vi "getData_v3.vi"() -> ()   [LabVIEW 2014]
uses:
  <vilib>/FPGAPlugInAG/cRIO-9039/niLvFpga_Open_cRIO-9039.vi
  <vilib>/Utility/error.llb/Error Cluster From Error Code.vi
  <vilib>/rvi/errors/niLvFpgaAdjustHostInterfaceError.vi
  <vilib>/Utility/file.llb/Write To Spreadsheet File (DBL).vi
  <vilib>/FPGAPlugInAG/cRIO-9039/niLvFpga_Close_cRIO-9039.vi
  <vilib>/rvi/interface/nirviOpenFPGA/nirviOpenFPGA.xnode
  FPGA Bitfiles/test0304_FPGATarget_test92159264_2zD5DwEAdGw.lvbitx
  <vilib>/rvi/interface/nirviMethod/nirviMethod.xnode
  <vilib>/rvi/interface/nirviCloseFPGA/nirviCloseFPGA.xnode
  <vilib>/FPGAPlugInAG/cRIO-9039/niLvFpga_ReadFifo_cRIO-9039.vi
  <vilib>/rvi/errors/niLvFpgaMergeErrorWithErrorCode.vi
panel:
  out "FIFO empty":bool
  out "Elements Remaining":u32=10000
  in  "Time_read":i32=10000
  out "message":string=" INSTRUCTIONS:\r\rNormal Use:  When using subVIs that incorporate the error in/error out (or error I/O) structure, place this handler where you want to inform the user of an error, typically at the end of the I/O data path, as the last action of the program.  If the error in error? is ERROR, the handler creates a message describing the error and its source.  If the type of dialog = 1 (default), the message is displayed to the user, who can only acknowedge it.  If the type = 2, the user can acknowledge the message or abort execution; aborting a program with active I/O is not recommended.  If the type = 0, no message is displayed; this is used to process the error programmatically, and the error out cluster elements are wired to individual terminals for that reason.  \r\rOther Use:\n\r\nlocal testing.  To test the error code of a subVI or function that does not have the error I/O structure, you can wire its error code and a source string to the local error code and error source inputs.  If error in error? indicates no error and error code is not equal to 0, the local code and source are substituted for the error in values, and error? is set TRUE (ERROR)."
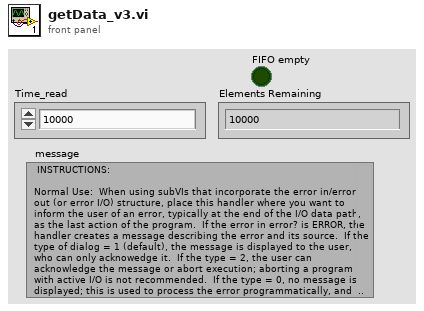
[diagram p1: front panel]
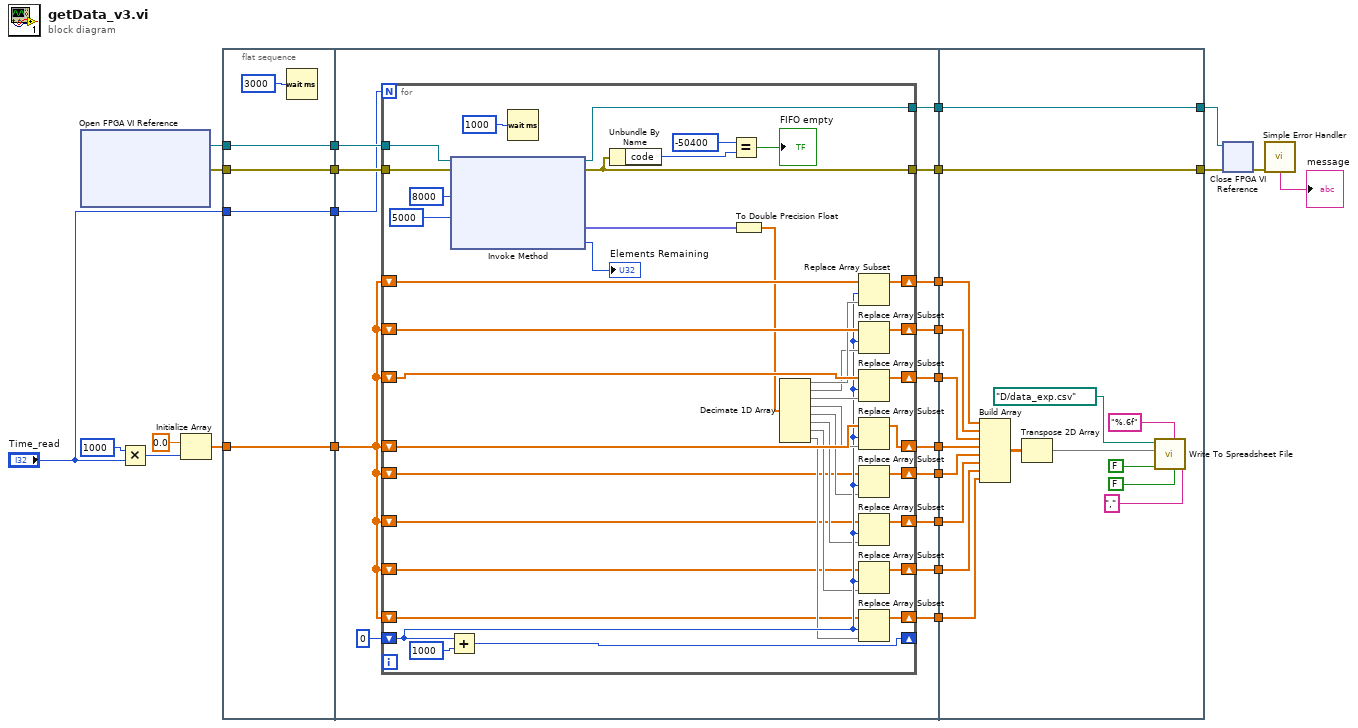
[diagram p0: block diagram]
diagram:
  n1 = xnode "Open FPGA VI Reference"() -> ("FPGA VI Reference Out"=w2:refnum<k20>, "error out"=w1:errorcluster)  [unwired: 2 in]
  n2 = Multiply(x=1000 ("y"), y="Time_read") -> (x*y=w18:i32)
  n3 = Initialize Array(0.0 ("element"), w18) -> (w22:dbl[])
  n4 = flat-sequence {
    tunnel: "Time_read" -> [w27]
    tunnel: w1 -> [w28]
    tunnel: w2 -> [w29]
    tunnel: w22 -> [w30]
    tunnel: [w30] -> w6
    tunnel: [w29] -> w5
    tunnel: [w28] -> w4
    tunnel: [w27] -> w3
    tunnel: [w42] -> w16
    tunnel: [w41] -> w15
    tunnel: [w40] -> w14
    tunnel: [w39] -> w13
    tunnel: [w38] -> w12
    tunnel: [w36] -> w11
    tunnel: [w35] -> w10
    tunnel: [w34] -> w9
    tunnel: [w33] -> w8
    tunnel: [w32] -> w7
    tunnel: w6 -> [w37]
    tunnel: w5 -> [w44]
    tunnel: w4 -> [w43]
    tunnel: w3 -> [w31]
    tunnel: w16 -> [w99]
    tunnel: w15 -> [w98]
    tunnel: w14 -> [w97]
    tunnel: [w102] -> w21
    tunnel: w13 -> [w102]
    tunnel: [w101] -> w20
    tunnel: w12 -> [w101]
    tunnel: w11 -> [w96]
    tunnel: w10 -> [w95]
    tunnel: w9 -> [w93]
    tunnel: w8 -> [w94]
    tunnel: w7 -> [w100]
    frame #0 {
      n5 = Wait (ms)(milliseconds to wait=u32 3000 ("y")) -> ()  [unwired: 1 out]
    }
    frame #1 {
      n6 = for {
        N: w31 -> [_]
        shift-right: [w83] -> _
        shift-left: 0 -> [w69]
        shift-right: [w72] -> w42
        shift-left: w37 -> [w81]
        shift-right: [w71] -> w41
        shift-left: w37 -> [w80]
        shift-right: [w70] -> w40
        shift-left: w37 -> [w79]
        shift-right: [w73] -> w32
        shift-left: w37 -> [w82]
        tunnel: w44 -> [w53]
        tunnel: w43 -> [w52]
        tunnel: [w48] -> w39
        tunnel: [w49] -> w38
        shift-right: [w63] -> w36
        shift-left: w37 -> [w64]
        shift-right: [w61] -> w35
        shift-left: w37 -> [w62]
        shift-right: [w60] -> w33
        shift-left: w37 -> [w59]
        shift-right: [w57] -> w34
        shift-left: w37 -> [w58]
        n7 = Add(x=w69, y=1000) -> (x+y=w83:i32)
        n8 = xnode "Invoke Method"("FPGA VI Reference In"=w53, "error in"=w52, "Number of Elements"=u32 8000, "Timeout (ms)"=5000) -> ("FPGA VI Reference Out"=w48:refnum<k20>, "error out"=w49:errorcluster, "Data"=w46:fxp<+/-,41,17>[], "Elements Remaining"=→"Elements Remaining":u32)
        n9 = Wait (ms)(milliseconds to wait=u32 1000 ("y")) -> ()  [unwired: 1 out]
        n10 = Unbundle By Name(w49) -> ("code"=w55:i32)
        n11 = Equal?(x=-50400 ("y"), y=w55) -> (x = y?=→"FIFO empty":bool)
        n12 = To Double Precision Float(number=w46) -> (double precision float=w78:dbl[])
        n13 = Decimate 1D Array(w78) -> (w77:dbl[], w76:dbl[], w75:dbl[], w74:dbl[], w68:dbl[], w67:dbl[], w66:dbl[], w65:dbl[])
        n14 = Replace Array Subset(array=w82, new element=w77, index=w69) -> (w73:dbl[])
        n15 = Replace Array Subset(array=w81, new element=w76, index=w69) -> (w72:dbl[])
        n16 = Replace Array Subset(array=w80, new element=w75, index=w69) -> (w71:dbl[])
        n17 = Replace Array Subset(array=w79, new element=w74, index=w69) -> (w70:dbl[])
        n18 = Replace Array Subset(array=w64, new element=w68, index=w69) -> (w63:dbl[])
        n19 = Replace Array Subset(array=w62, new element=w67, index=w69) -> (w61:dbl[])
        n20 = Replace Array Subset(array=w59, new element=w66, index=w69) -> (w60:dbl[])
        n21 = Replace Array Subset(array=w58, new element=w65, index=w69) -> (w57:dbl[])
      }
    }
    frame #2 {
      n22 = Build Array(w100, w99, w98, w97, w96, w95, w94, w93) -> (w86:dbl[][])
      n23 = Transpose 2D Array(2D array=w86) -> (transposed array=w91:dbl[][])
      n24 = call-poly <vilib>:"Write To Spreadsheet File.vi"("delimiter (\\t)"="," ("delimiter (\\t)"), "transpose? (no:F)"=FALSE, "format (%.3f)"="%.6f" ("format (%d)"), "append to file? (new file:F)"=FALSE, "2D data"=w91, "file path (dialog if empty)"=path "D:/data_exp.csv") -> ()  [unwired: 2 in, 1 out]
    }
  }
  n25 = xnode "Close FPGA VI Reference"("FPGA VI Reference In"=w21, "error in"=w20) -> ("error out"=w24:errorcluster)
  n26 = call <vilib>:"Simple Error Handler.vi"("error in (no error)"=w24) -> ("message"=→"message":string)  [unwired: 4 in, 4 out]
